vi "Hatch & Cargo Control.vi"   [LabVIEW 2018]
uses:
  <vilib>/Rock Robotics/WPI/ThirdParty/Phoenix-LabVIEW/Motor Controller/Controls/CTRE_Phoenix_MotorControl_NeutralMode.ctl
  <vilib>/Rock Robotics/WPI/ThirdParty/Phoenix-LabVIEW/Motor Controller/Controls/CTRE_Phoenix_MotorControl_ControlMode.ctl
  Infrastructure/RobotMap.vi
  Infrastructure/Constants.vi
  <vilib>/Rock Robotics/Network Tables/NT Read Number.vi
  Robot Global Data.vi
  <vilib>/Rock Robotics/WPI/ThirdParty/Phoenix-LabVIEW/Motor Controller/Get/CTRE_Phoenix_MotorController_GetOutputCurrent_Enhanced.vi
types:
  T1 = typedef "CTRE_Phoenix_MotorControl_NeutralMode.ctl" = enum8{"EEPROMSetting", "Override to Coast", "Override to Brake"}
  T2 = typedef "WPI_MotorControlDeviceRef.ctl" = cluster{"DeviceStatus":errorcluster, "Type":T3, "PWM":cluster{"PWM Channel":T4, "DeadBand":T5}, "CAN":cluster{"Device Number":u8, "SetOutput VI Ref":variant, "GetOutput VI Ref":variant, "Enable VI Ref":variant, "Disable VI Ref":variant, "Data":variant}, "Invert":bool, "DIO PWM":cluster{"PWM \"Enable\" Channel":T4, "DIOChannel":T6, "PWM Rate":dbl}}
  T3 = typedef "WPI_MotorControlType.ctl" = enum16{"PWM", "CAN", "DIO PWM"}
  T4 = typedef "FPGA_DIOPWMChannel.ctl" = enum8{"PWM 0", "PWM 1", "PWM 2", "PWM 3", "PWM 4", "PWM 5", "PWM 6", "PWM 7", "PWM 8", "PWM 9", "PWM MXP 0", "PWM MXP 1", "PWM MXP 2", "PWM MXP 3", "PWM MXP 4", "PWM MXP 5", "PWM MXP 6", "PWM MXP 7", "PWM MXP 8", "PWM MXP 9", "Invalid"}
  T5 = typedef "WPI_PWMDeadband.ctl" = cluster{"Name":string, "maxPositivePwm":i32, "minPositivePwm":i32, "centerPwm":i32, "maxNegativePwm":i32, "minNegativePwm":i32, "angularRange":u16}
  T6 = typedef "FPGA_DIOChannel.ctl" = enum8{"DIO 0", "DIO 1", "DIO 2", "DIO 3", "DIO 4", "DIO 5", "DIO 6", "DIO 7", "DIO 8", "DIO 9", "DIO MXP 0", "DIO MXP 1", "DIO MXP 2", "DIO MXP 3", "DIO MXP 4", "DIO MXP 5", "DIO MXP 6", "DIO MXP 7", "DIO MXP 8", "DIO MXP 9", "DIO MXP 10", "DIO MXP 11", "DIO MXP 12", "DIO MXP 13", "DIO MXP 14", "DIO MXP 15", "SPI Port CS1", "SPI Port CS2", "SPI Port CS3", "SPI Port MISO", "SPI Port MOSI", "Invalid"}
  T7 = cluster{"Cruise Velocity":i32, "Acceleration":i32}
  T8 = cluster{"P":dbl, "I":dbl, "D":dbl, "F":dbl, "I Zone":dbl}
  T9 = typedef "CTRE_Phoenix_MotorControl_ControlMode.ctl" = u16
  T10 = cluster{"Cargo Motor Value":dbl, "Hatch Setpoint":dbl}
  T11 = typedef "Joystick Controls.ctl" = cluster{"Driver Left Joystick X":dbl, "Driver Left Joystick Y":dbl, "Driver A Button":bool, "Driver B Button":bool, "Driver X Button":bool, "Driver Y Button":bool, "Driver Left Bumper":bool, "Driver Right Bumper":bool, "Driver View Button":bool, "Driver Menu Button":bool, "Driver Left Joystick Press":bool, "Driver Right Joystick Press":bool, "Driver Left Trigger":dbl, "Driver Right Joystick X":dbl, "Driver Right Joystick Y":dbl, "Driver Right Trigger":dbl, "Operator Left Joystick X":dbl, "Operator Left Joystick Y":dbl, "Operator A Button":bool, "Operator B Button":bool, "Operator X Button":bool, "Operator Y Button":bool, "Operator Left Bumper":bool, "Operator Right Bumper":bool, "Operator View Button":bool, "Operator Menu Button":bool, "Operator Left Joystick Press":bool, "Operator Right Joystick Press":bool, "Operator Left Trigger":dbl, "Operator Right Joystick X":dbl, "Operator Right Joystick Y":dbl, "Operator Right Trigger":dbl, "Driver D-Pad":i16, "Operator D-Pad":i16}
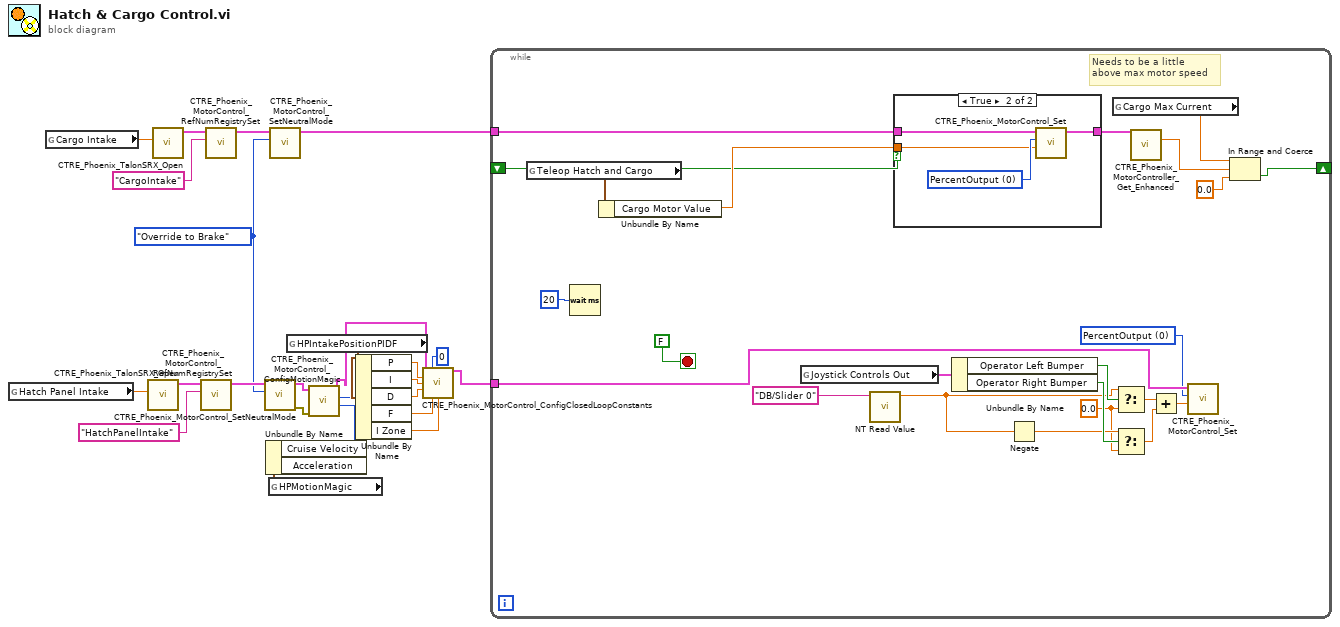
[diagram p0: block diagram]
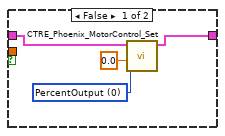
[diagram p2: hidden frame]
diagram:
  w16 = CTRE_Phoenix_MotorControl_NeutralMode."Override to Brake" ("Motor Control Neutral Mode")
  n1 = global read "RobotMap.vi" "Hatch Panel Intake"() -> (w21:dbl)
  n2 = global read "RobotMap.vi" "Cargo Intake"() -> (w22:dbl)
  n3 = call <vilib>:"CTRE_Phoenix_TalonSRX_Open.vi"("Device Number"=w21) -> ("CAN Talon SRX Ref"=w23:T2)  [unwired: 9 in, 1 out]
  n4 = call <vilib>:"CTRE_Phoenix_TalonSRX_Open.vi"("Device Number"=w22) -> ("CAN Talon SRX Ref"=w24:T2)  [unwired: 9 in, 1 out]
  n5 = call <vilib>:"CTRE_Phoenix_MotorControl_RefNumRegistrySet.vi"("refnum name"="HatchPanelIntake", "PhoenixMotorControlDevRef"=w23) -> ("PhoenixMotorControlDevRef"=w17:T2)  [unwired: 8 in, 1 out]
  n6 = call <vilib>:"CTRE_Phoenix_MotorControl_RefNumRegistrySet.vi"("refnum name"="CargoIntake", "PhoenixMotorControlDevRef"=w24) -> ("PhoenixMotorControlDevRef"=w18:T2)  [unwired: 8 in, 1 out]
  n7 = call <vilib>:"CTRE_Phoenix_MotorControl_SetNeutralMode.vi"("Motor Control Neutral Mode"=w16, "PhoenixMotorControlDevRef"=w17) -> ("error out"=w6:errorcluster, "PhoenixMotorControlDevRef"=w5:T2)  [unwired: 8 in]
  n8 = global read "Constants.vi" "HPMotionMagic"() -> (w3:T7)
  n9 = Unbundle By Name(w3) -> ("Cruise Velocity"=w2:i32, "Acceleration"=w1:i32)
  n10 = call <vilib>:"CTRE_Phoenix_MotorControl_SetNeutralMode.vi"("Motor Control Neutral Mode"=w16, "PhoenixMotorControlDevRef"=w18) -> ("PhoenixMotorControlDevRef"=w14:T2)  [unwired: 8 in, 1 out]
  n11 = global read "Constants.vi" "HPIntakePositionPIDF"() -> (w13:T8)
  n12 = call <vilib>:"CTRE_Phoenix_MotorControl_ConfigMotionMagic.vi"("error in (no error)"=w6, "Acceleration"=w1, "Cruise Velocity"=w2, "PhoenixMotorControlDevRef"=w5) -> ("PhoenixMotorControlDevRef"=w4:T2)  [unwired: 6 in, 1 out]
  n13 = Unbundle By Name(w13) -> ("P"=w12:dbl, "I"=w11:dbl, "D"=w10:dbl, "F"=w9:dbl, "I Zone"=w8:dbl)
  n14 = call <vilib>:"CTRE_Phoenix_MotorControl_ConfigClosedLoopConstants.vi"("PhoenixMotorControlDevRef"=w4, "slotIdx"=0, "P"=w12, "I"=w11, "D"=w10, "F"=w9, "I Zone"=w8) -> ("PhoenixMotorControlDevRef"=w15:T2)  [unwired: 7 in, 1 out]
  n15 = while {
    tunnel: w15 -> [w44]
    tunnel: w14 -> [w47]
    shift-right: [w28] -> _
    shift-left: _ -> [w25]
    stop <- FALSE stop-if-true
    w32 = 0.0 ("f")
    w31 = T9 0 items=["PercentOutput"=0, "Position"=1, "Velocity"=2, "Current"=3, "Follower"=5, "MotionProfile"=6, "MotionMagic"=7, "MotionProfileArc"=10, "Disabled"=15] ("Control Mode")
    # "Needs to be a little\nabove max motor speed"
    n16 = global read "Robot Global Data.vi" "Teleop Hatch and Cargo"() -> (w43:T10)
    n17 = Wait (ms)(milliseconds to wait=u32 20) -> ()  [unwired: 1 out]
    n18 = Unbundle By Name(w43) -> ("Cargo Motor Value"=w42:dbl)
    n19 = global read "Robot Global Data.vi" "Joystick Controls Out"() -> (w39:T11)
    n20 = call-poly <vilib>:"NT Read Value.vi"("Name"="DB/Slider 0") -> ("Numeric"=w35:dbl)  [unwired: 9 in, 1 out]
    n21 = case shown="True" w25 {
      tunnel: w47 -> [w51 w55]
      tunnel: w42 -> [_ w53]
      tunnel: [w50 w52] -> w30
      frame False {
        w48 = T9 0 items=["PercentOutput"=0, "Position"=1, "Velocity"=2, "Current"=3, "Follower"=5, "MotionProfile"=6, "MotionMagic"=7, "MotionProfileArc"=10, "Disabled"=15] ("Control Mode")
        n22 = call <vilib>:"CTRE_Phoenix_MotorControl_Set.vi"("Output"=0.0, "Control Mode"=w48, "PhoenixMotorControlDevRef"=w51) -> ("PhoenixMotorControlDevRef"=w50:T2)  [unwired: 7 in, 1 out]
      }
      frame True {
        w54 = T9 0 items=["PercentOutput"=0, "Position"=1, "Velocity"=2, "Current"=3, "Follower"=5, "MotionProfile"=6, "MotionMagic"=7, "MotionProfileArc"=10, "Disabled"=15] ("Control Mode")
        n23 = call <vilib>:"CTRE_Phoenix_MotorControl_Set.vi"("Output"=w53, "Control Mode"=w54, "PhoenixMotorControlDevRef"=w55) -> ("PhoenixMotorControlDevRef"=w52:T2)  [unwired: 7 in, 1 out]
      }
    }
    n24 = Unbundle By Name(w39) -> ("Operator Left Bumper"=w40:bool, "Operator Right Bumper"=w41:bool)
    n25 = Negate(x=w35) -> (-x=w34:dbl)
    n26 = global read "Constants.vi" "Cargo Max Current"() -> (w26:dbl)
    n27 = Select(t=w35, s=w40, f=w32) -> (s? t:f=w36:dbl)
    n28 = Select(t=w34, s=w41, f=w32) -> (s? t:f=w37:dbl)
    n29 = call-poly <vilib>:"CTRE_Phoenix_MotorController_Get_Enhanced.vi"("PhoenixMotorControlDevRef"=w30) -> ("Output Current"=w29:dbl)  [unwired: 12 in, 2 out]
    n30 = Add(x=w36, y=w37) -> (x+y=w38:dbl)
    n31 = call <vilib>:"CTRE_Phoenix_MotorControl_Set.vi"("Output"=w38, "Control Mode"=w31, "PhoenixMotorControlDevRef"=w44) -> ()  [unwired: 7 in, 2 out]
    n32 = In Range and Coerce(upper limit=w26, x=w29, lower limit=0.0) -> (In Range?=w28:bool)  [unwired: 1 out]
  }
